vi "WM_CAP - ARGB to BGRA.vi"(7 "ARGB":u8[](array[numeric]), 13 "Image Depth":u16) -> (8 "BGRA":u8[](array[numeric]))   [LabVIEW 2022 SP3]
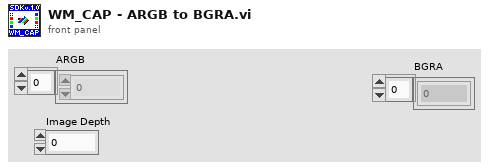
[diagram p1: front panel]
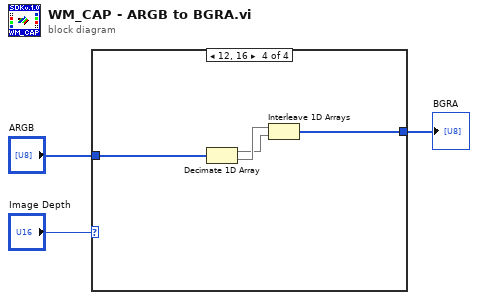
[diagram p0: block diagram]
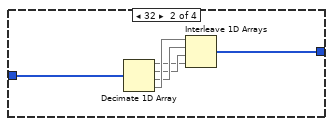
[diagram p3: hidden frame]
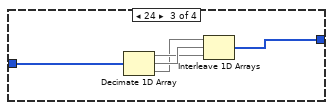
[diagram p4: hidden frame]
diagram:
  n1 = case shown="12, 16" "Image Depth" {
    tunnel: "ARGB" -> [w4 w6 w13 w17]
    tunnel: [w4 w5 w12 w16] -> w2
    frame 8, Default {
    }
    frame 32 {
      n2 = Decimate 1D Array(w6) -> (w7:u8[], w8:u8[], w9:u8[], w10:u8[])
      n3 = Interleave 1D Arrays(w10, w9, w8, w7) -> (w5:u8[])
    }
    frame 24 {
      n4 = Decimate 1D Array(w13) -> (w14:u8[], w15:u8[], w11:u8[])
      n5 = Interleave 1D Arrays(w11, w15, w14) -> (w12:u8[])
    }
    frame 12, 16 {
      n6 = Decimate 1D Array(w17) -> (w18:u8[], w19:u8[])
      n7 = Interleave 1D Arrays(w19, w18) -> (w16:u8[])
    }
  }
  "BGRA" <- w2
